vi "find row in array.vi"(8 "error in (no error)":errorcluster, 9 "parameter name":string, 10 "limit values":string[][](array[string])) -> (0 "error out":errorcluster, 2 "row":string[](array[string]))   [LabVIEW 2018]
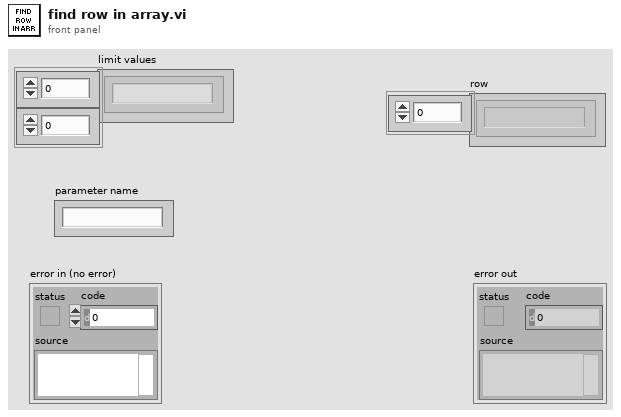
[diagram p1: front panel]
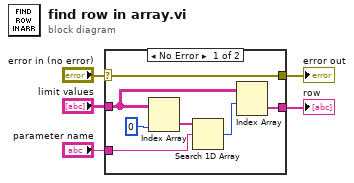
[diagram p0: block diagram]
diagram:
  n1 = case shown="No Error" "error in (no error)" {
    selector: "error in (no error)" -> [w12 w13]
    tunnel: [w12 w13] -> w4
    tunnel: "limit values" -> [w7 _]
    tunnel: "parameter name" -> [w8 _]
    tunnel: [w6 _] -> w1
    frame No Error {
      n2 = Index Array(array=w7, index (col)=0 ("disabled index (col)")) -> (element=w9:string[])  [unwired: 1 in]
      n3 = Search 1D Array(1D array=w9, element=w8) -> (index of element=w10:i32)  [unwired: 1 in]
      n4 = Index Array(array=w7, index (row)=w10) -> (element=w6:string[])  [unwired: 1 in]
    }
    frame Error {
    }
  }
  "error out" <- w4
  "row" <- w1
